vi "Intake Arm Controller.vi"(8 "error in":errorcluster) -> ()   [LabVIEW 2020]
doc: "This VI executes continuously carrying out the current operation and responding to updates or new operations. It will often contain the timing or control code that is difficult to place directly in TeleOp. This VI generally opens all sensors and motors and isolates the rest of the robot code from knowing how the operations are carried out."
uses:
  <vilib>/Rock Robotics/WPI/Framework/Completion Status.ctl
  Intake Arm Setpoints.ctl
  Intake Arm Operations.ctl
  <vilib>/Rock Robotics/WPI/SafetyOutput/WPI_SafetyOutputConfigMenu.ctl
  <vilib>/Rock Robotics/WPI/Solenoid/WPI_SolenoidChannel.ctl
  <vilib>/Rock Robotics/WPI/Solenoid/WPI_SolenoidValue.ctl
  <vilib>/Rock Robotics/WPI/Solenoid/WPI_SolenoidOpenDouble.vi
  <vilib>/Rock Robotics/WPI/Solenoid/WPI_SolenoidSetEnum.vi
  <vilib>/Rock Robotics/Network Tables/NT Write Number.vi
panel:
  in  "Interactive Values":T1
  out "Current\nCmd":string
  in  "Buttons":cluster{"Execute Cmd":bool, "Abort Cmd":bool}
  out "Command Timing":cluster{"Start Time (ms)":u32, "Iterations":i32}
  out "Status":T3
  # "Tip: It may be helpful to observe inputs and sensor values.\nYou may also want to display tuning or debugging controls."
  # "Interactive Command: You may fill in the settings for a command\nand schedule it with the Execute button. You can observe and abort\nany command while fine tuning the code for the controller."
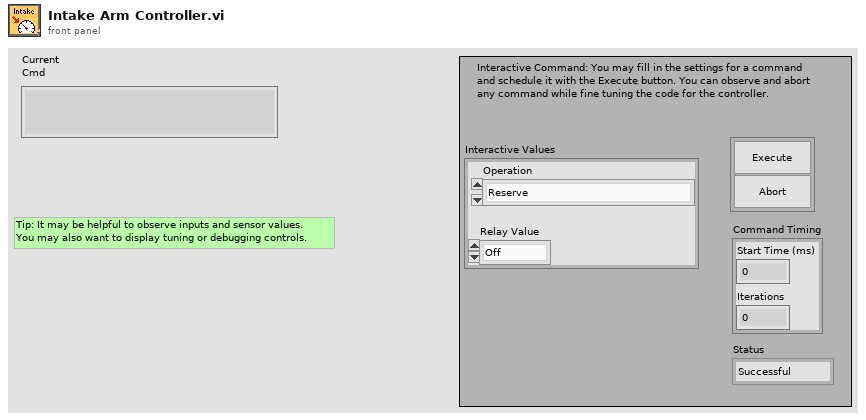
[diagram p1: front panel]
types:
  T1 = typedef "Intake Arm Setpoints.ctl" = cluster{"Operation":T2, "Relay Value":enum16{"Off", "On", "Forward", "Reverse"}}
  T2 = typedef "Intake Arm Operations.ctl" = enum16{"Reserve", "Read Current", "Immediate", "Intake Arm Immediate", "Up", "Down"}
  T3 = typedef "Completion Status.ctl" = enum16{"Successful", "Aborted", "Incomplete"}
  T4 = typedef "WPI_SolenoidValue.ctl" = enum16{"Off", "On", "Forward", "Reverse"}
  T5 = typedef "WPI_SolenoidChannel.ctl" = enum8{"Solenoid 0", "Solenoid 1", "Solenoid 2", "Solenoid 3", "Solenoid 4", "Solenoid 5", "Solenoid 6", "Solenoid 7", "Solenoid 8", "Solenoid 9", "Solenoid 10", "Solenoid 11", "Solenoid 12", "Solenoid 13", "Solenoid 14", "Solenoid 15", "Invalid"}
  T6 = typedef "WPI_SafetyOutputConfigMenu.ctl" = enum16{"Enable", "Disable"}
  T7 = typedef "WPI_SolenoidDevRef.ctl" = cluster{"DevStatus":errorcluster, "Pneumatics Control Module":u8, "Forward Solenoid Channel":T5, "Reverse Solenoid Channel":T5}
  T8 = typedef "Command Status Info.ctl" = cluster{"Name":string, "Status":T3, "notifier out":T9}
  T9 = typedef "Completion Notifier.ctl" = refnum<notifier>
  T10 = cluster{"Current Command":T1, "Command Timing":cluster{"Start Time (ms)":u32, "Iterations":i32}, "Command Arguments":cluster{"Command Info":T8, "Description":string, "Default Command":T1, "queue out":refnum<queue>, "Subsystem Name":string}}
  T11 = cluster{u32, "Relay Value":enum16{"Off", "On", "Forward", "Reverse"}}
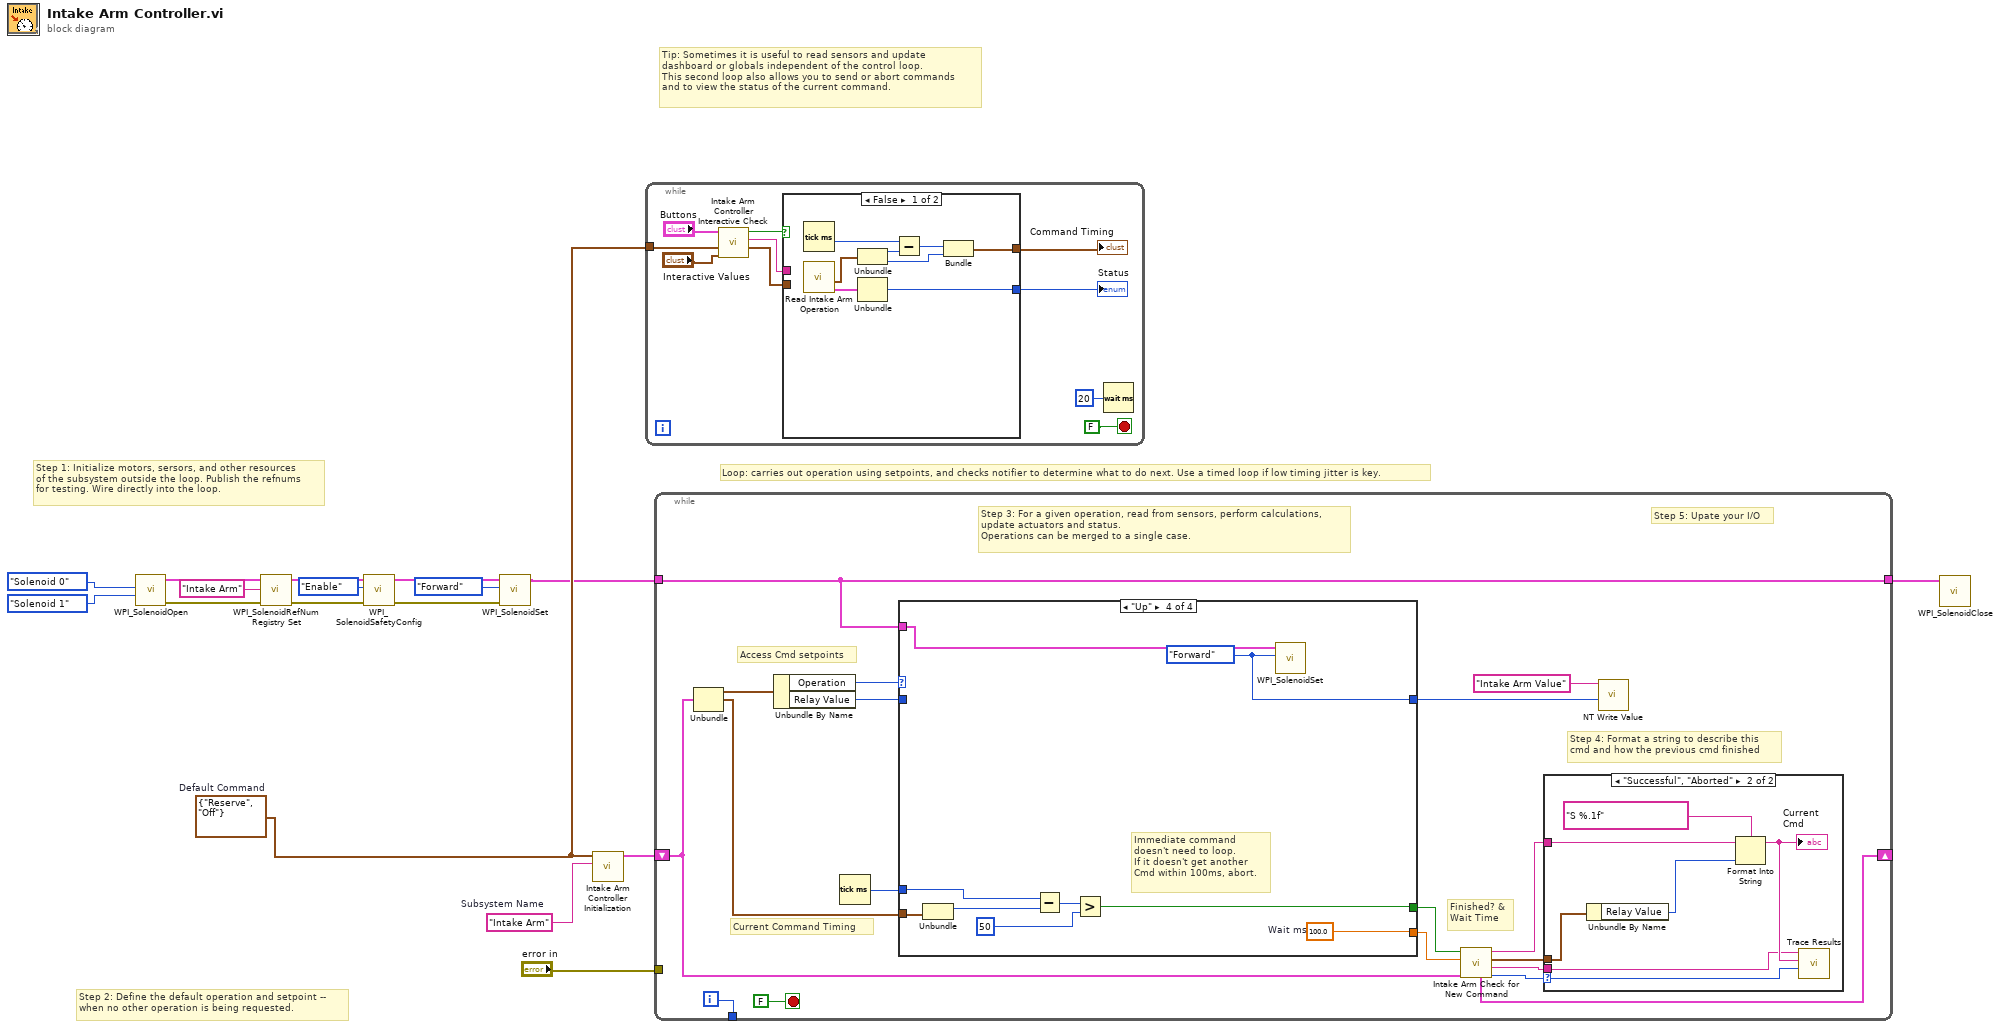
[diagram p0: block diagram]
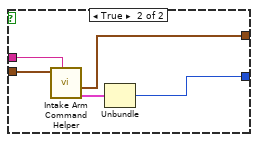
[diagram p2: hidden frame]
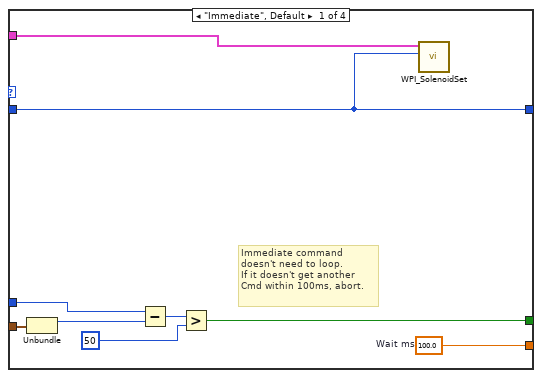
[diagram p4: hidden frame]
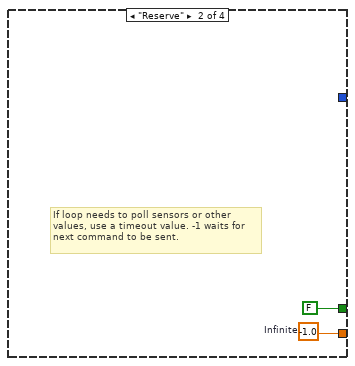
[diagram p5: hidden frame]
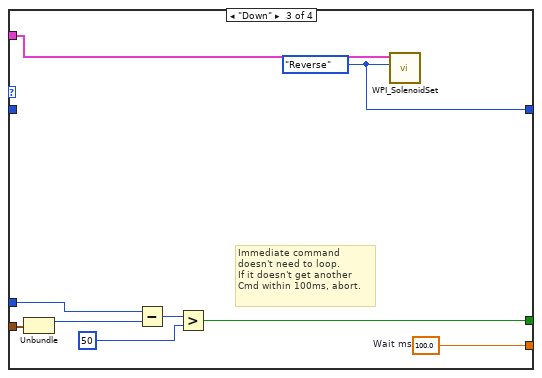
[diagram p6: hidden frame]
diagram:
  w14 = T1 {"Operation"=enum."Reserve", "Relay Value"=enum."Off"}  # Default Command
  w15 = "Intake Arm"  # Subsystem Name
  # "Tip: Sometimes it is useful to read sensors and update\ndashboard or globals independent of the control loop.\nThis second loop also allows you to send or abort commands\nand to view the status of the current command."
  # "Step 2: Define the default operation and setpoint --\nwhen no other operation is being requested."
  # "Step 1: Initialize motors, sersors, and other resources\nof the subsystem outside the loop. Publish the refnums\nfor testing. Wire directly into the loop."
  # "Loop: carries out operation using setpoints, and checks notifier to determine what to do next. Use a timed loop if low timing jitter is key."
  n1 = call-poly <vilib>:"WPI_SolenoidOpen.vi"("Reverse Solenoid Channel"=WPI_SolenoidChannel."Solenoid 1", "Forward Solenoid Channel"=WPI_SolenoidChannel."Solenoid 0") -> ("error out"=w12:errorcluster, "SolenoidDevRef"=w11:T7)  [unwired: 8 in]
  n2 = call <vilib>:"WPI_SolenoidRefNum Registry Set.vi"("error in (no error)"=w12, "refnum name"="Intake Arm", "SolenoidDevRef"=w11) -> ("error out"=w10:errorcluster, "SolenoidDevRef"=w9:T7)  [unwired: 7 in]
  n3 = call <vilib>:"WPI_SolenoidSafetyConfig.vi"("error in (no error)"=w10, "mode"=WPI_SafetyOutputConfigMenu."Enable", "SolenoidDevRef"=w9) -> ("error out"=w8:errorcluster, "SolenoidDevRef"=w7:T7)  [unwired: 7 in]
  n4 = call-poly <vilib>:"WPI_SolenoidSet.vi"("error in (no error)"=w8, "Value"=WPI_SolenoidValue."Forward", "SolenoidDevRef"=w7) -> ("SolenoidDevRef"=w2:T7)  [unwired: 7 in, 1 out]
  n5 = call "Intake Arm Controller Initialization.vi"("Subsystem Name"=w15, "Default Command"=w14) -> ("Current Command"=w16:T10)  [unwired: 9 in]
  n6 = while {
    tunnel: w14 -> [w24]
    stop <- FALSE stop-if-true
    n7 = call "Intake Arm Controller Interactive Check.vi"("Interactive Command in"="Interactive Values", "Default Command"=w24, "Buttons"="Buttons") -> ("Interactive Command out"=w21:T1, "Trace String"=w22:string, "Schedule"=w23:bool)  [unwired: 6 in]
    n8 = case shown="False" w23 {
      tunnel: [w35 w40] -> w20
      tunnel: w21 -> [_ w38]
      tunnel: [w31 w36] -> w19
      tunnel: w22 -> [_ w39]
      frame False {
        n9 = Tick Count (ms)() -> (millisecond timer value=w30:u32)
        n10 = call "Read Intake Arm Operation.vi"() -> ("Command Info"=w28:T8, "SubSystem Data"=w29:T1)  [unwired: 9 in, 1 out]
        n11 = Unbundle(w29) -> ("Operation"=w34:T2, "Relay Value"=w32:enum16{"Off", "On", "Forward", "Reverse"})
        n12 = Unbundle(w28) -> ("Status"=w35:T3)  [unwired: 2 out]
        n13 = Subtract(x=w30, y=w34) -> (x-y=w33:u32)
        n14 = Bundle(w33, "Relay Value"=w32) -> (w31:T11)  [unwired: 1 in]
      }
      frame True {
        n15 = call "Intake Arm Command Helper.vi"("Description"=w39, "SubSystem Data"=w38) -> ("Command Info Out"=w37:T8, "Command Timing"=w36:cluster{"Start Time (ms)":u32, "Iterations":i32})  [unwired: 7 in, 1 out]
        n16 = Unbundle(w37) -> ("Status"=w40:T3)  [unwired: 2 out]
      }
    }
    "Status" <- w20
    "Command Timing" <- w19
    n17 = Wait (ms)(milliseconds to wait=u32 20) -> ()  [unwired: 1 out]
  }
  n18 = while {
    shift-right: [w53] -> _
    shift-left: w16 -> [w46]
    tunnel: [w57] -> _
    tunnel: "error in" -> [_]
    tunnel: w2 -> [w41]
    tunnel: [w41] -> w13
    i -> [w57]
    stop <- FALSE stop-if-true
    # "Step 5: Upate your I/O"
    # "Step 4: Format a string to describe this\ncmd and how the previous cmd finished"
    # "Current Command Timing"
    # "Access Cmd setpoints"
    # "Finished? &\nWait Time"
    # "Step 3: For a given operation, read from sensors, perform calculations,\nupdate actuators and status.\nOperations can be merged to a single case."
    n19 = Unbundle(w46) -> ("Current Command"=w56:T1, "Command Timing"=w54:cluster{"Start Time (ms)":u32, "Iterations":i32})  [unwired: 1 out]
    n20 = Unbundle By Name(w56) -> ("Operation"=w45:T2, "Relay Value"=w44:enum16{"Off", "On", "Forward", "Reverse"})
    n21 = Tick Count (ms)() -> (millisecond timer value=w55:u32)
    n22 = case shown="\"Up\"" w45 {
      tunnel: [w74 w76 w77 w86] -> w51
      tunnel: [w68 FALSE ("ignore previous (F)") w78 w87] -> w52
      tunnel: w54 -> [w70 _ w79 w89]
      tunnel: w55 -> [w69 _ w80 w88]
      tunnel: w41 -> [w67 _ w85 w94]
      tunnel: w44 -> [w66 _ _ _]
      tunnel: [w66 _ w84 w93] -> w43
      frame "Immediate", Default {
        w74 = 100.0  # Wait ms
        # "Immediate command\ndoesn't need to loop.\nIf it doesn't get another\nCmd within 100ms, abort."
        n23 = Unbundle(w70) -> ("Start Time (ms)"=w73:u32)  [unwired: 1 out]
        n24 = Subtract(x=w69, y=w73) -> (x-y=w72:u32)
        n25 = Greater?(x=w72, y=u8 50 ("Left Motor")) -> (0:w68:bool)
        n26 = call-poly <vilib>:"WPI_SolenoidSet.vi"("Value"=w66, "SolenoidDevRef"=w67) -> ()  [unwired: 8 in, 2 out]
      }
      frame "Reserve" {
        w76 = -1.0  # Infinite
        # "If loop needs to poll sensors or other\nvalues, use a timeout value. -1 waits for\nnext command to be sent."
      }
      frame "Down" {
        w77 = 100.0  # Wait ms
        w84 = WPI_SolenoidValue."Reverse" ("Value")
        # "Immediate command\ndoesn't need to loop.\nIf it doesn't get another\nCmd within 100ms, abort."
        n27 = Unbundle(w79) -> ("Start Time (ms)"=w83:u32)  [unwired: 1 out]
        n28 = Subtract(x=w80, y=w83) -> (x-y=w82:u32)
        n29 = Greater?(x=w82, y=u8 50 ("Left Motor")) -> (0:w78:bool)
        n30 = call-poly <vilib>:"WPI_SolenoidSet.vi"("Value"=w84, "SolenoidDevRef"=w85) -> ()  [unwired: 8 in, 2 out]
      }
      frame "Up" {
        w86 = 100.0  # Wait ms
        w93 = WPI_SolenoidValue."Forward" ("Value")
        # "Immediate command\ndoesn't need to loop.\nIf it doesn't get another\nCmd within 100ms, abort."
        n31 = Unbundle(w89) -> ("Start Time (ms)"=w92:u32)  [unwired: 1 out]
        n32 = Subtract(x=w88, y=w92) -> (x-y=w91:u32)
        n33 = Greater?(x=w91, y=u8 50 ("Left Motor")) -> (0:w87:bool)
        n34 = call-poly <vilib>:"WPI_SolenoidSet.vi"("Value"=w93, "SolenoidDevRef"=w94) -> ()  [unwired: 8 in, 2 out]
      }
    }
    n35 = call "Intake Arm Check for New Command.vi"("Current Command"=w46, "Wait time (ms)"=w51, "Finished?"=w52) -> ("Completion"=w47:T3, "Subsystem Name"=w48:string, "Current Command"=w49:T1, "Initial Trace String"=w50:string, "NextCommand"=w53:T10)  [unwired: 4 in]
    n36 = case shown="\"Successful\", \"Aborted\"" w47 {
      selector: w47 -> [_ w65]
      tunnel: w50 -> [_ w62]
      tunnel: w49 -> [_ w63]
      tunnel: w48 -> [_ w60]
      frame "Incomplete", Default {
        # "Continuing current command"
      }
      frame "Successful", "Aborted" {
        # "Report and setup for next command"
        n37 = Unbundle By Name(w63) -> ("Relay Value"=w59:enum16{"Off", "On", "Forward", "Reverse"})
        n38 = Format Into String(format string="S %.1f", initial string=w62, w59) -> (resulting string=w61:string)  [unwired: 1 in, 1 out]
        "Current\nCmd" <- w61
        n39 = call <vilib>:"Trace Results.vi"("Status of previous command"=w65, "Description"=w61, "Subsystem"=w60) -> ()  [unwired: 9 in]
      }
    }
    n40 = call-poly <vilib>:"NT Write Value.vi"("Numeric"=w43, "Name"="Intake Arm Value") -> ()  [unwired: 9 in, 1 out]
  }
  n41 = call <vilib>:"WPI_SolenoidClose.vi"("SolenoidDevRef"=w13) -> ()  [unwired: 10 in, 1 out]
